vi "DSF.Engine.Execution.Transfer.RT FIFO.Data.To.vi"(8 "error in (no error)":errorcluster, 11 "Transfer in":refnum<class "DSF.Engine.Execution.Transfer.lvclass">) -> (0 "error out":errorcluster, 2 "Transfer Data":T1 {"Buffer Descriptor"."address" format="%016x"; "Buffer Descriptor"."size" format="%d bytes"}, 3 "Transfer out":refnum<class "DSF.Engine.Execution.Transfer.lvclass">)   [LabVIEW 2016, in "DSF.Engine.lvlib" / "DSF.Engine.Execution.Transfer.lvclass"]
uses:
  DSF.Engine.Execution.Transfer.lvclass
  DSF.Engine.Execution.Transfer.RT FIFO Data.ctl
  DSF.Engine.Execution.Transfer.lvclass/DSF.Engine.Execution.Transfer.ctl
  Submodules/Memory/Source/Classes/Pointer/Memory.Pointer.lvclass/Memory.Pointer.ctl
  Submodules/Memory/Source/Classes/Pointer/Memory.Pointer.Get Address.vi
  Submodules/Memory/Source/Classes/Pointer/Memory.Pointer.Get Size.vi
  Buffer/DSF.Engine.Memory.Buffer.lvclass
  C:/Git/SourceTree/DSF/Source/Submodules/Memory/Source/Classes/Pointer/Memory.Pointer.lvclass
  Submodules/Memory/Source/Classes/Pointer/Memory.Pointer.lvclass
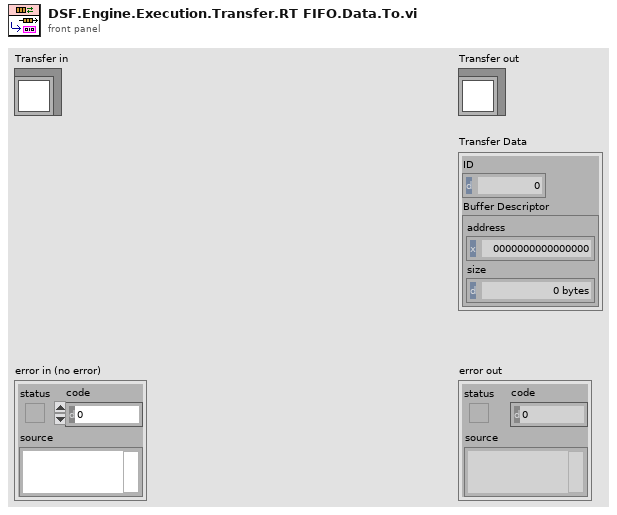
[diagram p1: front panel]
types:
  T1 = typedef "DSF.Engine.lvlib/DSF.Engine.Execution.Transfer.lvclass/DSF.Engine.Execution.Transfer.RT FIFO Data.ctl" = cluster{"ID":i32, "Buffer Descriptor":cluster{"address":u64, "size":u64}}
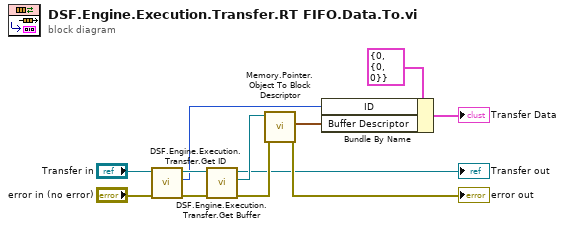
[diagram p0: block diagram]
diagram:
  n1 = call "DSF.Engine.Execution.Transfer.Get ID.vi"("error in (no error)"="error in (no error)", "Transfer in"="Transfer in") -> ("error out"=w9:errorcluster, "id"=w7:i32, "Transfer out"=w10:refnum<class "DSF.Engine.Execution.Transfer.lvclass">)  [unwired: 7 in]
  n2 = call "DSF.Engine.Execution.Transfer.Get Buffer.vi"("error in (no error)"=w9, "Transfer in"=w10) -> ("error out"=w5:errorcluster, "Buffer"=w3:refnum<class "DSF.Engine.Memory.Buffer.lvclass">, "Transfer out"=→"Transfer out":refnum<class "DSF.Engine.Execution.Transfer.lvclass">)  [unwired: 7 in]
  n3 = call "Memory.Pointer.Object To Block Descriptor.vi"("error in (no error)"=w5, "pointer in"=w3) -> ("error out"=→"error out":errorcluster, "block descriptor"=w6:cluster{"address":u64, "size":u64})  [unwired: 7 in, 1 out]
  n4 = Bundle By Name(cluster=T1 {"ID"=0, "Buffer Descriptor"={"address"=0, "size"=0}} ("Transfer Data"), "ID"=w7, "Buffer Descriptor"=w6) -> (→"Transfer Data":T1)
